vi "test_Name.vi"(8 "error in (no error)":errorcluster, 11 "TestCase in":refnum<class "[Test Case] Strip path.lvclass">) -> (0 "error out":errorcluster, 3 "TestCase out":refnum<class "[Test Case] Strip path.lvclass">)   [LabVIEW 2016, in "Tests.lvlib" / "[Test Case] Strip path.lvclass"]
uses:
  [Test Case] Strip path.lvclass
  [Test Case] Strip path.lvclass/[Test Case] Strip path.ctl
  <vilib>/addons/_JKI Toolkits/VI Tester/TestCase.llb/TestCase.lvclass
  classes/File Transfer Behavior/File Transfer Behavior.lvclass
  C:/Program Files (x86)/National Instruments/LabVIEW 2016/vi.lib/addons/_JKI Toolkits/VI Tester/TestCase.llb/TestCase.lvclass
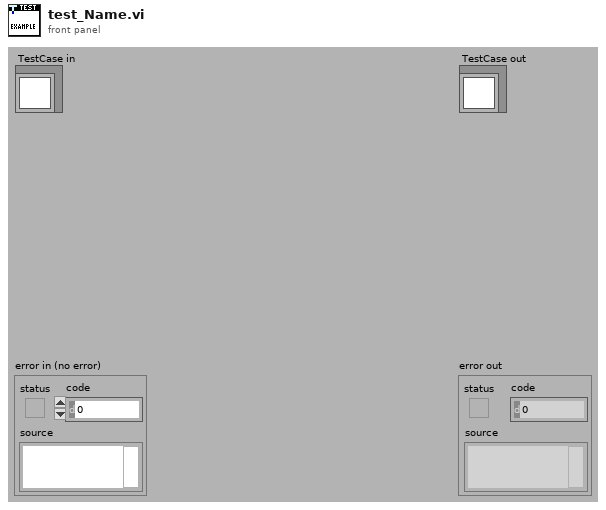
[diagram p1: front panel]
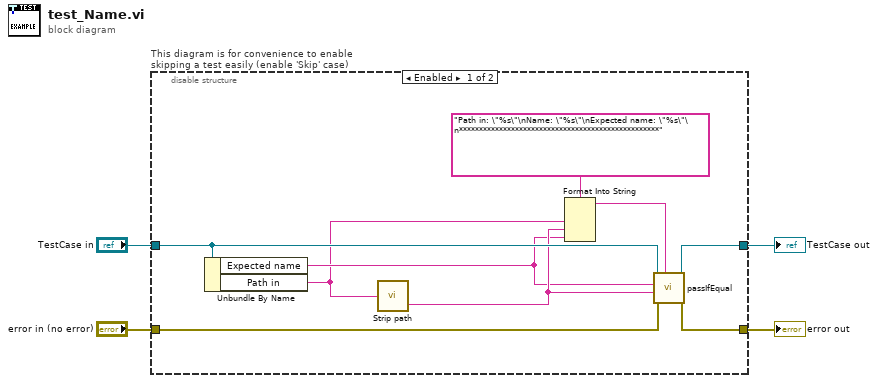
[diagram p0: block diagram]
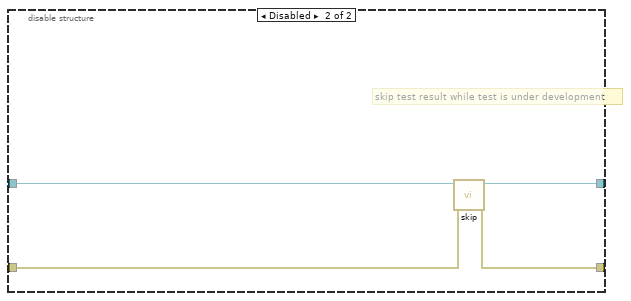
[diagram p2: hidden frame]
diagram:
  n1 = disable-structure "This diagram is for convenience to enable skipping a test easily (enable 'Skip' case)" shown="Enabled" {
    disable-tunnel: "TestCase in" -> [w10 w17]
    disable-tunnel: [w13 w15] -> w1
    disable-tunnel: [w12 w16] -> w3
    disable-tunnel: "error in (no error)" -> [w11 w14]
    frame Enabled {
      n2 = Unbundle By Name(w10) -> ("Expected name"=w6:string, "Path in"=w5:string)
      n3 = call "Strip path.vi"("Path"=w5) -> ("Name"=w8:string)  [unwired: 2 in, 1 out]
      n4 = Format Into String(format string="Path in: \"%s\"\nName: \"%s\"\nExpected name: \"%s\"\n**************************************************", w5, w8, w6) -> (resulting string=w7:string)  [unwired: 2 in, 1 out]
      n5 = call-dynamic "passIfEqual.vi"("custom report message (\"\")"=w7, "error in (no error)"=w11, "y"=w8, "x"=w6, "TestCase in"=w10) -> ("error out"=w12:errorcluster, "TestCase out"=w13:refnum<class "[Test Case] Strip path.lvclass">)  [unwired: 5 in]
    }
    frame Disabled {
      # "skip test result while test is under development"
      n6 = call <vilib>:"skip.vi"("error in (no error)"=w14, "TestCase in"=w17) -> ("error out"=w16:errorcluster, "TestCase out"=w15:refnum<class "[Test Case] Strip path.lvclass">)  [unwired: 8 in]
    }
  }
  "error out" <- w3
  "TestCase out" <- w1
